vi "cluster1.vi"() -> ()   [LabVIEW 2016]
panel:
  out "String":string
  out "element":dbl
  in  "Array":dbl[](array[numeric])
  in  "Cluster":T1
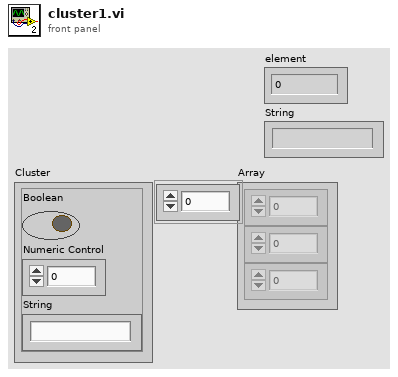
[diagram p1: front panel]
types:
  T1 = cluster{"Boolean":bool, "Numeric Control":dbl, "String":string}
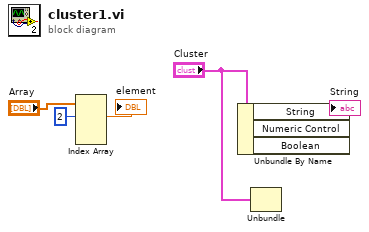
[diagram p0: block diagram]
diagram:
  n1 = Index Array(array="Array", index #1=2 ("index")) -> (element #1=→"element":dbl)  [unwired: 3 in, 3 out]
  n2 = Unbundle By Name("Cluster") -> ("String"=→"String":string)  [unwired: 2 out]
  n3 = Unbundle("Cluster") -> ()  [unwired: 3 out]
